vi "Basic Output demo.vi"() -> ()   [LabVIEW 2013]
panel:
  out "value":T1(array[cluster])
  in  "stop":bool
  out "Output (VKeys)":u8[](array[ring])
  out "Output (Virtual Keys)":i32[](array[numeric])
  out "mouse info":T2={"Axis Info 2"={"Horizontal"=123, "Vertical"=469, "Scrolling"=0}, "button 1"=FALSE, "button 2"=FALSE, "button 3"=FALSE, "button 4"=FALSE}
  in  "Input":T3(array[ring])
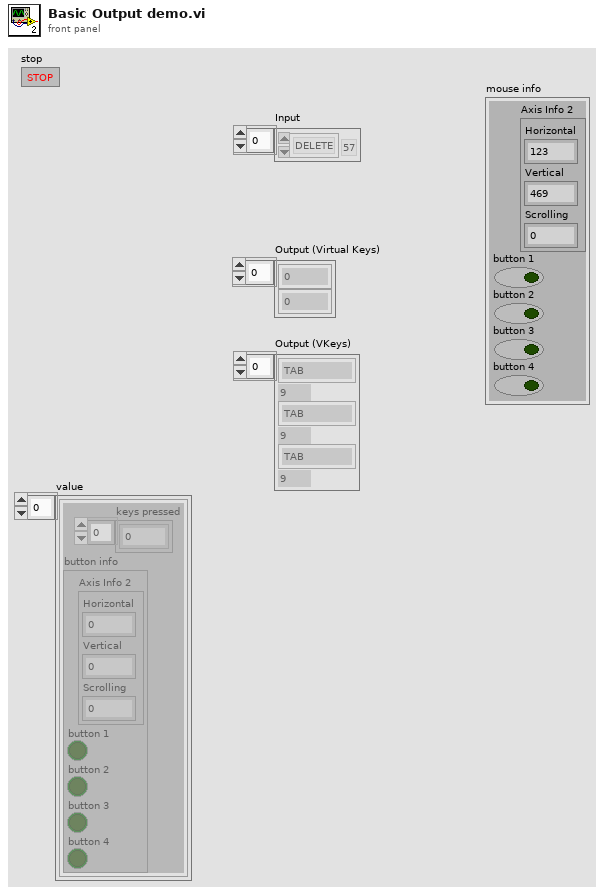
[diagram p1: front panel]
types:
  T1 = cluster{"keys pressed":enum16{"0", "1", "2", "3", "4", "5", "6", "7", "8", "9", "A", "B", "C", "D", "E", "F", "G", "H", "I", "J", "K", "L", "M", "N", "O", "P", "Q", "R", "S", "T", "U", "V", "W", "X", "Y", "Z", "F1", "F2", "F3", "F4", "F5", "F6", "F7", "F8", "F9", "F10", "F11", "F12", "F13", "F14", "F15", "ADD", "BACK", "BACKSLASH", "CAPITAL", "COMMA", "DECIMAL", "DELETE", "DIVIDE", "DOWN", "END", "EQUALS", "ESCAPE", "GRAVE (`)", "HOME", "INSERT", "LBRACKET", "LCONTROL", "LEFT", "L ALT", "LSHIFT", "LWIN", "MINUS", "MULTIPLY", "NEXT", "NUMLOCK", "NUMPAD_0", "NUMPAD_1", "NUMPAD_2", "NUMPAD_3", "NUMPAD_4", "NUMPAD_5", "NUMPAD_6", "NUMPAD_7", "NUMPAD_8", "NUMPAD_9", "PAUSE", "PERIOD", "PRIOR (PG UP)", "RBRACKET", "RCONTROL", "RETURN", "RIGHT", "R ALT", "RSHIFT", "RWIN", "SCROLL", "SEMICOLON", "SLASH", "SPACE", "SUBTRACT", "TAB", "UP", "ENTER (num pad)", "' (quote)"}[], "button info":cluster{"Axis Info 2":cluster{"Horizontal":i32, "Vertical":i32, "Scrolling":i32}, "button 1":bool, "button 2":bool, "button 3":bool, "button 4":bool}}[]
  T2 = cluster{"Axis Info 2":cluster{"Horizontal":i32, "Vertical":i32, "Scrolling":i32}, "button 1":bool, "button 2":bool, "button 3":bool, "button 4":bool}
  T3 = enum16{"0", "1", "2", "3", "4", "5", "6", "7", "8", "9", "A", "B", "C", "D", "E", "F", "G", "H", "I", "J", "K", "L", "M", "N", "O", "P", "Q", "R", "S", "T", "U", "V", "W", "X", "Y", "Z", "F1", "F2", "F3", "F4", "F5", "F6", "F7", "F8", "F9", "F10", "F11", "F12", "F13", "F14", "F15", "ADD", "BACK", "BACKSLASH", "CAPITAL", "COMMA", "DECIMAL", "DELETE", "DIVIDE", "DOWN", "END", "EQUALS", "ESCAPE", "GRAVE (`)", "HOME", "INSERT", "LBRACKET", "LCONTROL", "LEFT", "L ALT", "LSHIFT", "LWIN", "MINUS", "MULTIPLY", "NEXT", "NUMLOCK", "NUMPAD_0", "NUMPAD_1", "NUMPAD_2", "NUMPAD_3", "NUMPAD_4", "NUMPAD_5", "NUMPAD_6", "NUMPAD_7", "NUMPAD_8", "NUMPAD_9", "PAUSE", "PERIOD", "PRIOR (PG UP)", "RBRACKET", "RCONTROL", "RETURN", "RIGHT", "R ALT", "RSHIFT", "RWIN", "SCROLL", "SEMICOLON", "SLASH", "SPACE", "SUBTRACT", "TAB", "UP", "ENTER (num pad)", "' (quote)"}[]
  T4 = cluster{"button info":cluster{"Axis Info 2":cluster{"Horizontal":i32, "Vertical":i32, "Scrolling":i32}, "button 1":bool, "button 2":bool, "button 3":bool, "button 4":bool}}
  T5 = cluster{" Key":u8, "Action":enum16{"Press", "Up", "Down"}, "Delay (ms)":u32}
  T6 = enum16{"big-endian, network order", "native, host order", "little-endian"}
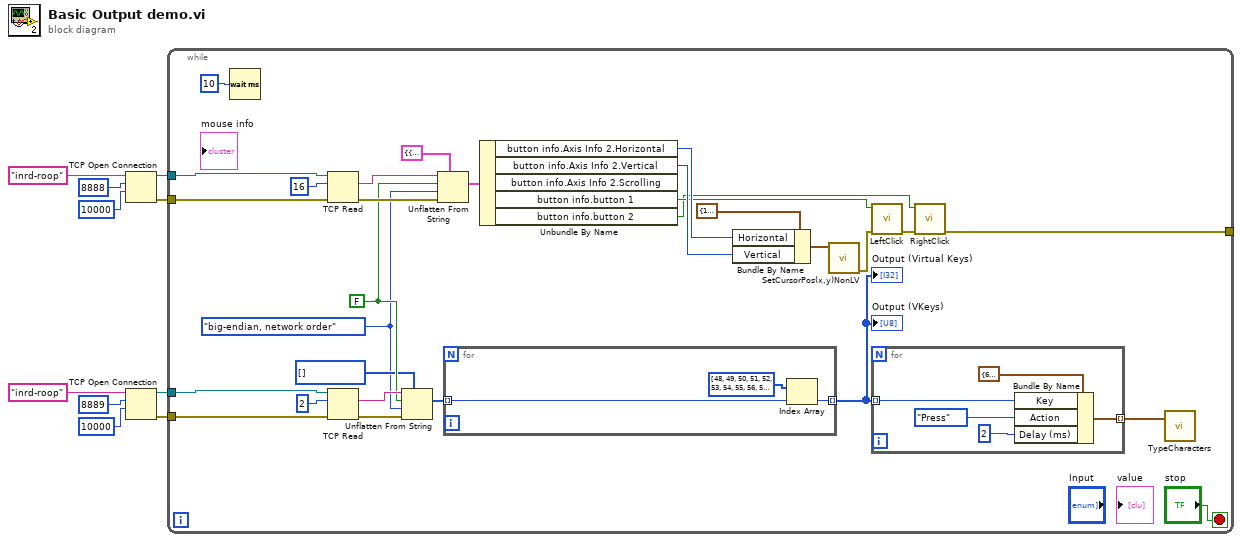
[diagram p0: block diagram]
diagram:
  n1 = TCP Open Connection(address="inrd-roop", remote port or service name=u16 8888, timeout ms (60000)=10000) -> (connection ID=w9:refnum<k5>, error out=w8:errorcluster)  [unwired: 2 in]
  n2 = TCP Open Connection(address="inrd-roop", remote port or service name=u16 8889, timeout ms (60000)=10000) -> (connection ID=w2:refnum<k5>, error out=w1:errorcluster)  [unwired: 2 in]
  n3 = while {
    tunnel: w9 -> [w38]
    tunnel: w8 -> [w37]
    tunnel: w2 -> [w24]
    tunnel: w1 -> [w23]
    tunnel: [w11] -> _
    stop <- "stop" stop-if-true
    w21 = T3 [] items=["0", "1", "2", "3", "4", "5", "6", "7", "8", "9", "A", "B", "C", "D", "E", "F", "G", "H", "I", "J", "K", "L", "M", "N", "O", "P", "Q", "R", "S", "T", "U", "V", "W", "X", "Y", "Z", "F1", "F2", "F3", "F4", "F5", "F6", "F7", "F8", "F9", "F10", "F11", "F12", "F13", "F14", "F15", "ADD", "BACK", "BACKSLASH", "CAPITAL", "COMMA", "DECIMAL", "DELETE", "DIVIDE", "DOWN", "END", "EQUALS", "ESCAPE", "GRAVE (`)", "HOME", "INSERT", "LBRACKET", "LCONTROL", "LEFT", "L ALT", "LSHIFT", "LWIN", "MINUS", "MULTIPLY", "NEXT", "NUMLOCK", "NUMPAD_0", "NUMPAD_1", "NUMPAD_2", "NUMPAD_3", "NUMPAD_4", "NUMPAD_5", "NUMPAD_6", "NUMPAD_7", "NUMPAD_8", "NUMPAD_9", "PAUSE", "PERIOD", "PRIOR (PG UP)", "RBRACKET", "RCONTROL", "RETURN", "RIGHT", "R ALT", "RSHIFT", "RWIN", "SCROLL", "SEMICOLON", "SLASH", "SPACE", "SUBTRACT", "TAB", "UP", "ENTER (num pad)", "' (quote)"] ("keys pressed")
    w22 = FALSE ("data includes array or string size? (T)")
    w20 = T6."big-endian, network order" ("byte order (0:big-endian, network order)")
    n4 = Wait (ms)(milliseconds to wait=u32 10) -> ()  [unwired: 1 out]
    n5 = TCP Read(connection ID=w38, bytes to read=16, error in (no error)=w37) -> (data out=w35:string, error out=w36:errorcluster)  [unwired: 2 in, 1 out]
    n6 = TCP Read(connection ID=w24, bytes to read=2, error in (no error)=w23) -> (data out=w26:string, error out=w25:errorcluster)  [unwired: 2 in, 1 out]
    n7 = Unflatten From String(type=w21, binary string=w26, data includes array or string size? (T)=w22, byte order (0:big-endian, network order)=w20, error in (no error)=w25) -> (value=w19:T3)  [unwired: 2 out]
    n8 = Unflatten From String(type=T4 {"button info"={"Axis Info 2"={"Horizontal"=0, "Vertical"=0, "Scrolling"=0}, "button 1"=FALSE, "button 2"=FALSE, "button 3"=FALSE, "button 4"=FALSE}}, binary string=w35, data includes array or string size? (T)=w22, byte order (0:big-endian, network order)=w20, error in (no error)=w36) -> (value=w18:T4)  [unwired: 2 out]
    n9 = for {
      tunnel: w19 -> [w41] mode=indexing
      tunnel: [w40] -> w28 mode=indexing
      n10 = Index Array(array=i32[] [48, 49, 50, 51, 52, 53, 54, 55, 56, 57, 65, 66, 67, 68, 69, 70, 71, 72, 73, 74, 75, 76, 77, 78, 79, 80, 81, 82, 83, 84, 85, 86, 87, 88, 89, 90, 112, 113, 114, 115, 116, 117, 118, 119, 120, 121, 122, 123, 124, 125, 126, 107, 8, 220, 20, 188, 110, 46, 111, 40, 35, 187, 27, 192, 36, 45, 219, 162, 37, 18, 16, 91, 189, 106, 34, 144, 96, 97, 98, 99, 100, 101, 102, 103, 104, 105, 19, 190, 33, 221, 163, 13, 39, 165, 161, 92, 145, 186, 191, 32, 109, 9, 38, 13, 222], index=w41) -> (element=w40:i32)
    }
    "Output (Virtual Keys)" <- w28
    "Output (VKeys)" <- w28
    n11 = Unbundle By Name(w18) -> ("button info.Axis Info 2.Horizontal"=w17:i32, "button info.Axis Info 2.Vertical"=w16:i32, "button info.button 1"=w15:bool, "button info.button 2"=w13:bool)  [unwired: 1 out]
    n12 = Bundle By Name(cluster=cluster{"Horizontal":i32, "Vertical":i32} {"Horizontal"=100, "Vertical"=100} ("RelativePosition"), "Horizontal"=w17, "Vertical"=w16) -> (w30:cluster{"Horizontal":i32, "Vertical":i32})
    n13 = call "SetCursorPos(x,y)NonLV.vi"("RelativePosition"=w30) -> ("error out"=w14:errorcluster)  [unwired: 9 in, 1 out]
    n14 = call "LeftClick.vi"("Error in (no error)"=w14, "Click?"=w15) -> ("Error out"=w12:errorcluster)  [unwired: 9 in]
    n15 = for {
      tunnel: w28 -> [w47] mode=indexing
      tunnel: [w45] -> w29 mode=indexing
      n16 = Bundle By Name(cluster=T5 {" Key"=65, "Action"=enum."Press", "Delay (ms)"=10} ("Cluster"), "Key"=w47, "Action"=enum16{"Press", "Up", "Down"}."Press", "Delay (ms)"=u32 2) -> (w45:T5)
    }
    n17 = call "RightClick.vi"("Error in (no error)"=w12, "Click?"=w13) -> ("Error out"=w11:errorcluster)  [unwired: 9 in]
    n18 = call "TypeCharacters.vi"("Key Array"=w29) -> ()  [unwired: 2 in]
  }
